vi "ScanDelay_FTIR_GetSpectrum_Aligning.vi"(0 "Cancel? External":refnum<vi>, 1 "% averaged (external)":refnum<vi>, 2 "Binned interferogram (external)":refnum<vi>, 3 "Python refnum in":refnum<k35>, 5 "Refresh alignment":bool=TRUE, 7 "Acquisition cycle (external)":refnum<vi>, 9 "Delay calibration\n          factor":dbl=2.403, 10 "Python error in":errorcluster, 11 "Subtract\ndelay (ps)":dbl, 12 "Acquisitions per interferogram":i32=20, 13 "Time per\nacquisition (s)":dbl=0.235, 14 "Sampling rate":dbl=250000.0, 15 "Extract envelope":bool=TRUE) -> (4 "Output spectrum":dbl[][](array[numeric]), 6 "Python error out":errorcluster)   [LabVIEW 2021]
uses:
  Control_GetSpectrum_Aligning.ctl
  <vilib>/DAQmx/read.llb/DAQmx Read (Analog 2D DBL NChan NSamp).vi
  <vilib>/DAQmx/miscellaneous.llb/DAQmx Fill In Error Info.vi
panel:
  out "DAQmx error":errorcluster={"status"=FALSE, "code"=200012, "source"="DAQmx Control Task.vi:3900001"}
  out "Time per\nloop (ms)":dbl=251.0
  in  "Save interferograms\n(interferograms.txt)":bool
  in  "Alignment order":i32=4
  out "Own python session":bool
  out "Refnum errors":errorcluster
  out "Spectrum (amplitude)":cluster{dbl[], dbl[]}[](graph)
  out "Spectrum (phase)":cluster{dbl[], dbl[]}(graph)
  out "Interferogram (aligned)":cluster{dbl, dbl}[](graph)
  out "% averaged":dbl=100.0
  out "Acquisition cycle":dbl[][](graph)
  in  "Halt acquisition":bool
  out "Python module path":path=path "C:/Users/mnopl/Desktop/Software/LabVIEW/ScanDelay/scandelay.py"
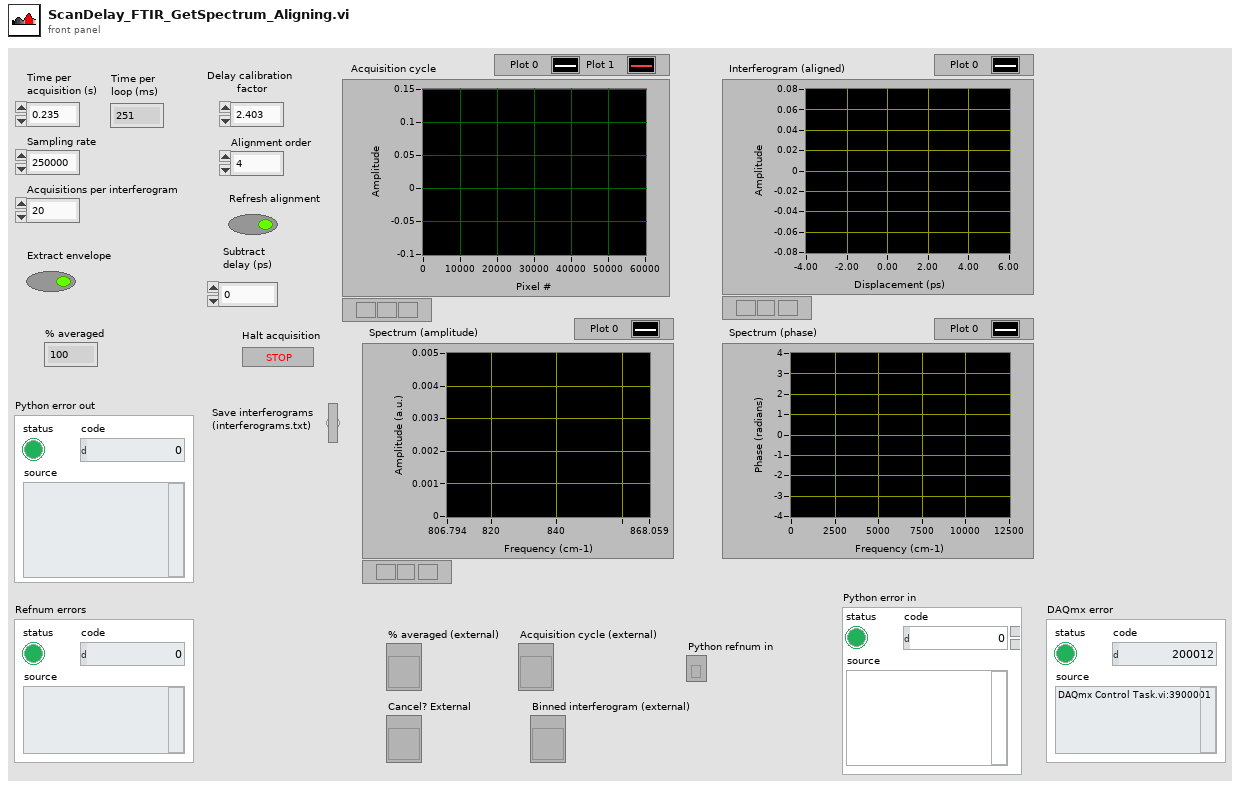
[diagram p1: front panel]
types:
  T1 = typedef "Control_GetSpectrum_Aligning.ctl" = enum16{"Acquire Interferograms", "Prepare DAQ task", "Align Interferograms", "Compute Spectrum", "Done"}
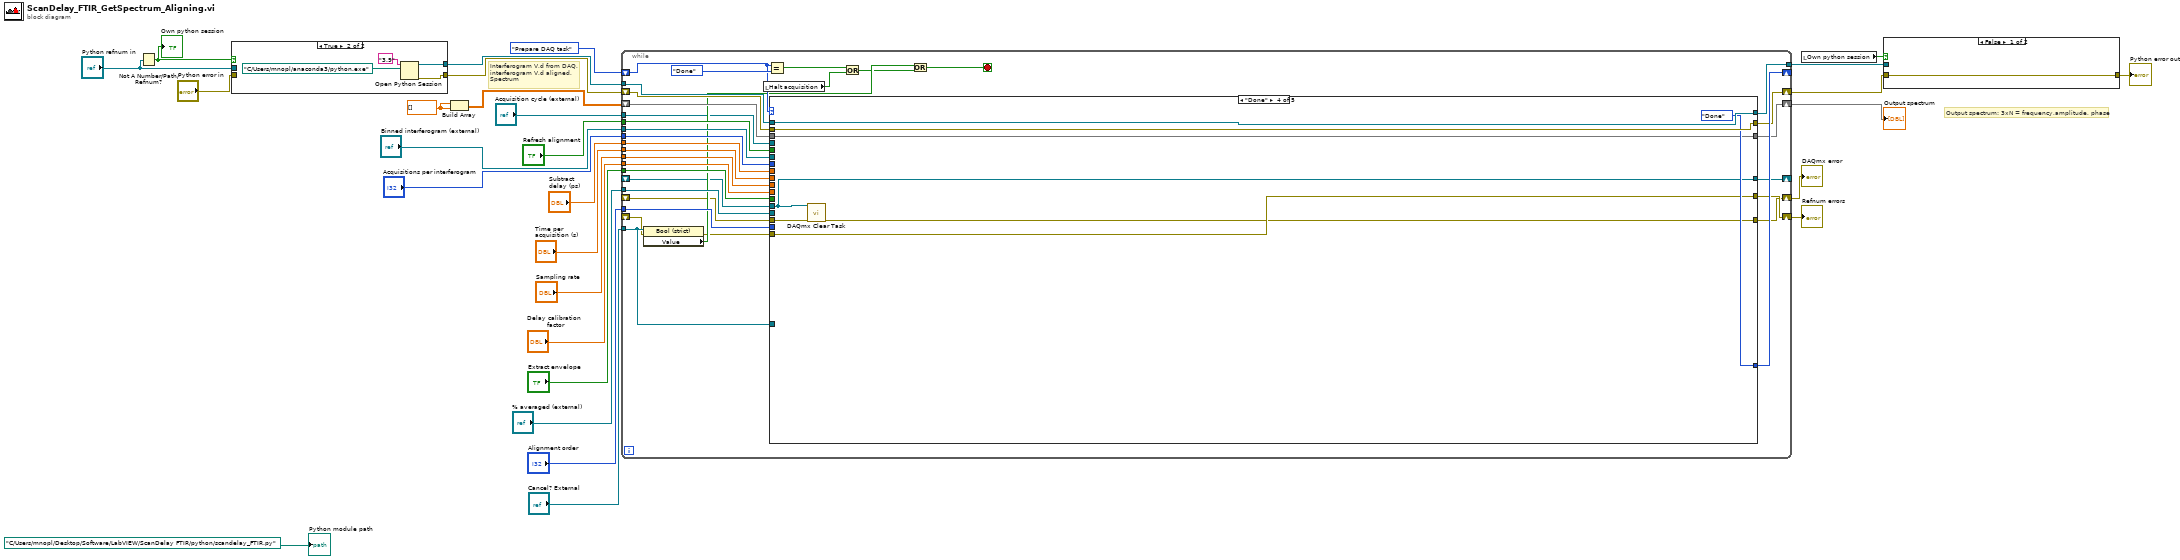
[diagram p0: block diagram]
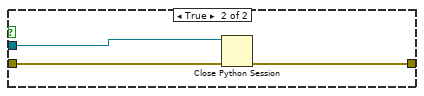
[diagram p2: hidden frame]
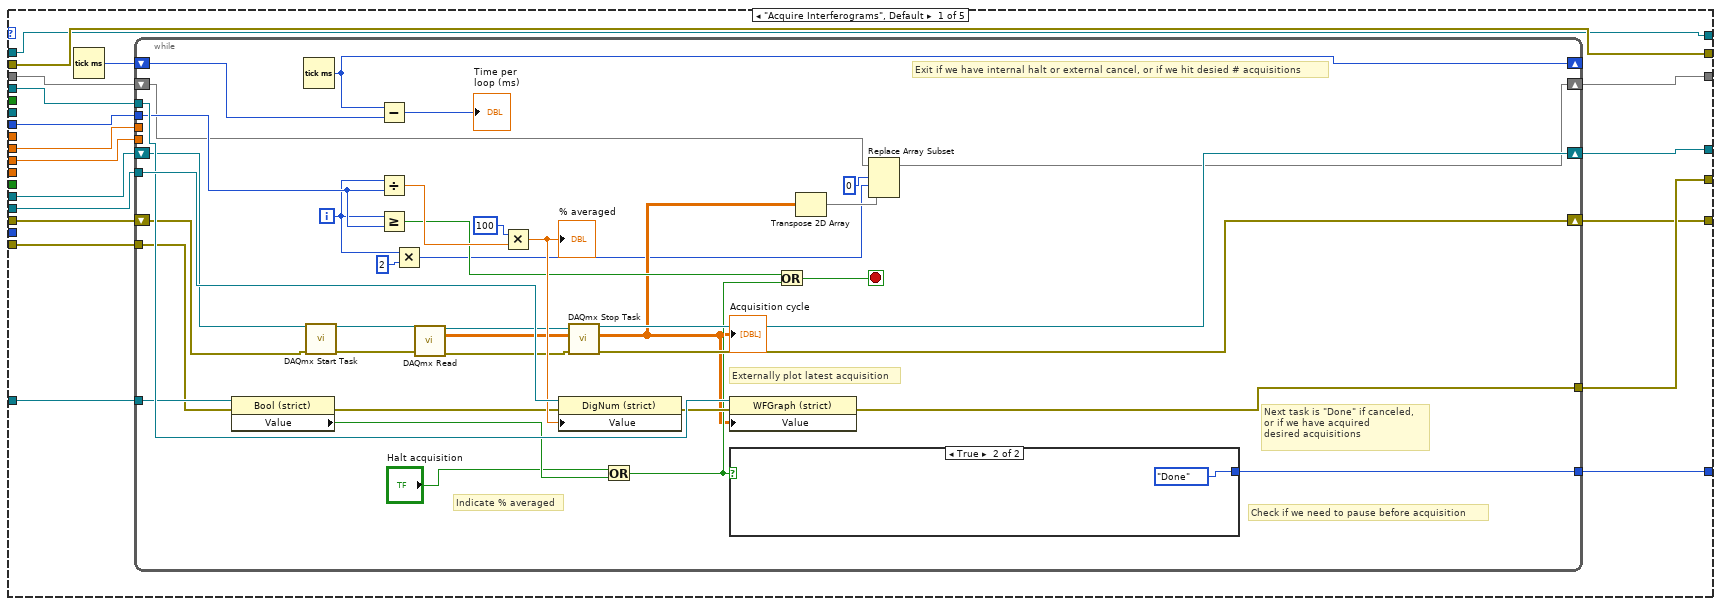
[diagram p4: hidden frame]
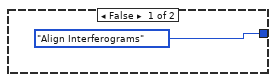
[diagram p5: hidden frame]
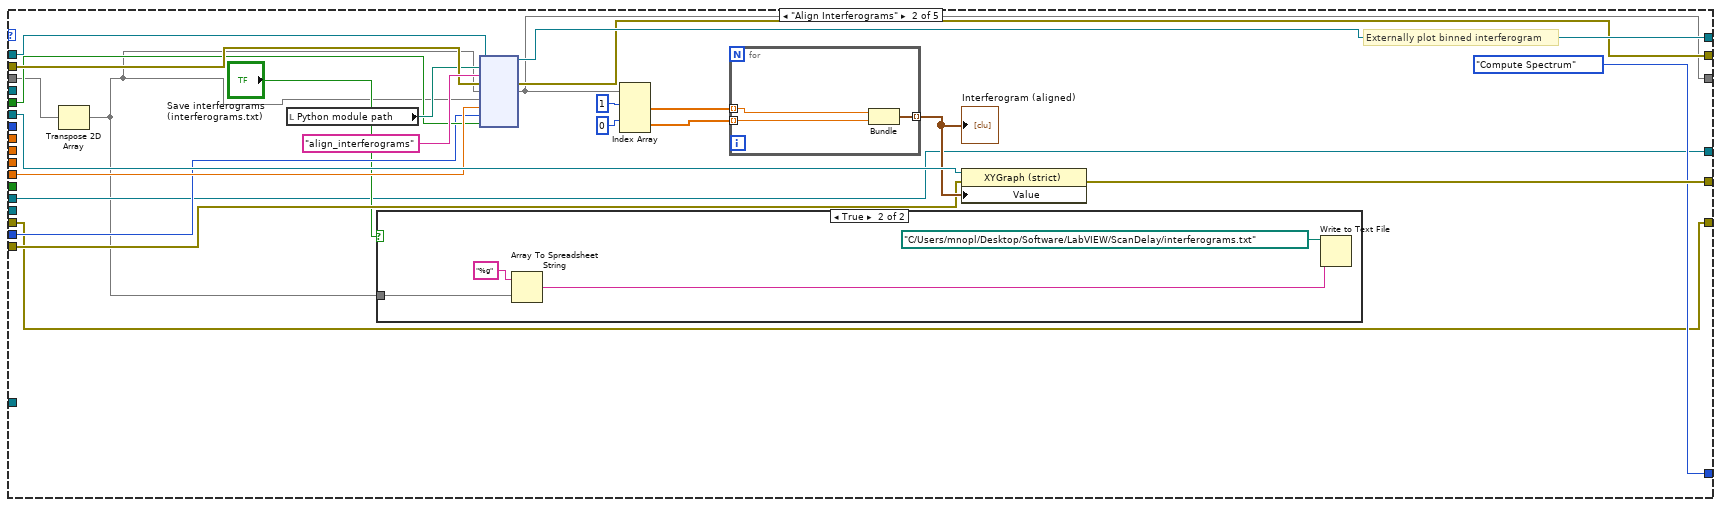
[diagram p6: hidden frame]
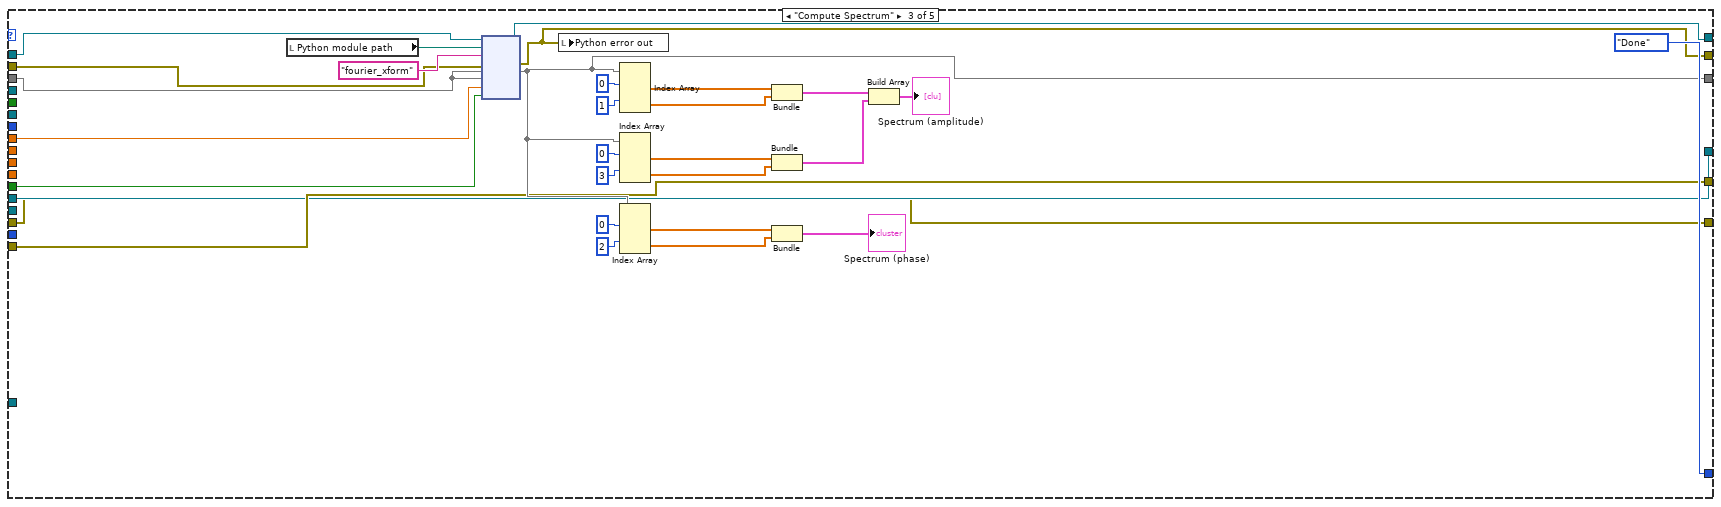
[diagram p8: hidden frame]
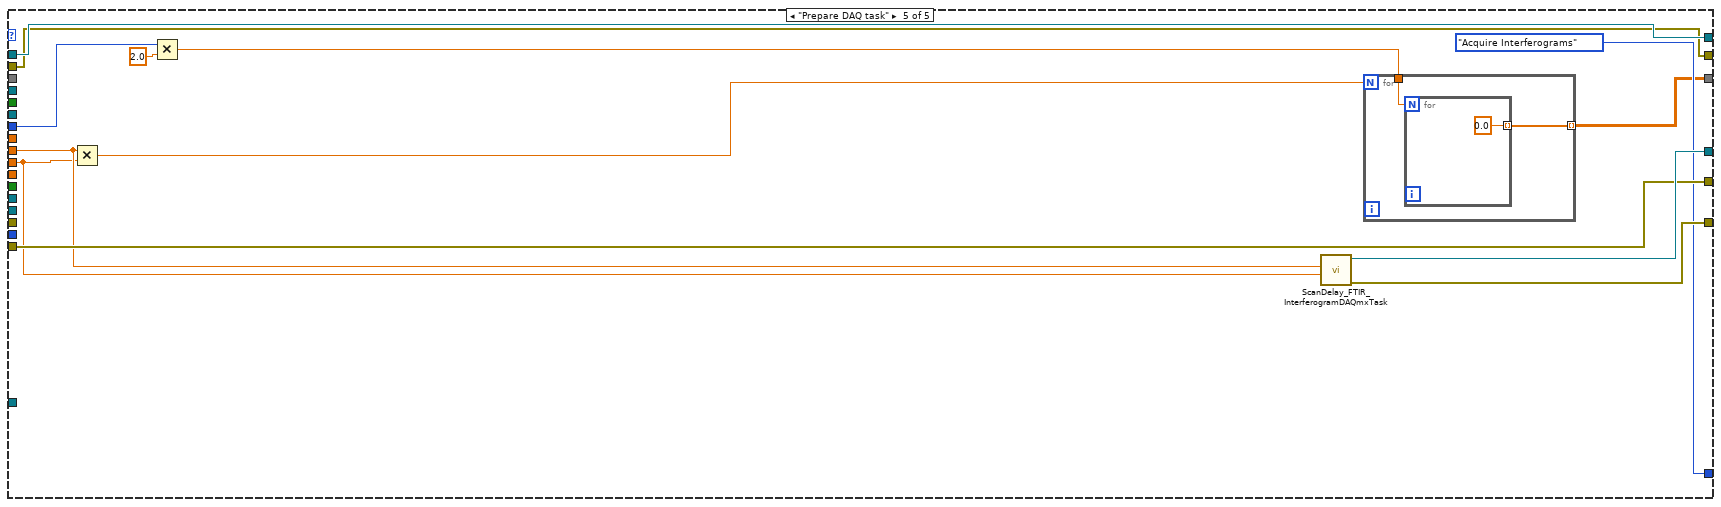
[diagram p9: hidden frame]
diagram:
  w17 = dbl[] []
  # "Output spectrum: 3xN = frequency,amplitude, phase"
  # "Interferogram V,d from DAQ,\ninterferogram V,d aligned,\nSpectrum"
  n1 = Not A Number/Path/Refnum?(number/path/refnum="Python refnum in") -> (NaN/Path/Refnum?=w7:bool)
  "Own python session" <- w7
  n2 = case shown="True" w7 {
    tunnel: [w30 w32] -> w11
    tunnel: [w29 w31] -> w10
    tunnel: "Python refnum in" -> [w30 _]
    tunnel: "Python error in" -> [w29 _]
    frame False {
    }
    frame True {
      n3 = Open Python Session(python version="3.9", python path=path "C:/Users/mnopl/anaconda3/python.exe") -> (session out=w32:refnum<k35>, error out=w31:errorcluster)  [unwired: 1 in]
    }
  }
  n4 = Build Array(w17, w17) -> (w4:dbl[][])
  n5 = while {
    shift-right: [w49] -> w16
    shift-left: w4 -> [w67]
    tunnel: w11 -> [w66]
    tunnel: "Acquisition cycle (external)" -> [w39]
    tunnel: "Sampling rate" -> [w64]
    tunnel: "Time per\nacquisition (s)" -> [w63]
    tunnel: "Delay calibration\n          factor" -> [w62]
    tunnel: "% averaged (external)" -> [w61]
    tunnel: "Cancel? External" -> [w42]
    tunnel: "Acquisitions per interferogram" -> [w60]
    shift-right: [w59] -> _
    shift-left: Control_GetSpectrum_Aligning."Prepare DAQ task" -> [w50]
    tunnel: "Subtract\ndelay (ps)" -> [w58]
    tunnel: [w55] -> w18
    shift-right: [w54] -> w15
    shift-left: w10 -> [w65]
    tunnel: "Extract envelope" -> [w53]
    shift-right: [w52] -> w13
    shift-left: _ -> [w40]
    tunnel: "Binned interferogram (external)" -> [w51]
    tunnel: "Refresh alignment" -> [w48]
    tunnel: "Alignment order" -> [w47]
    shift-right: [w37] -> w1
    shift-left: _ -> [w35]
    shift-right: [w38] -> _
    shift-left: _ -> [w36]
    stop <- w44 stop-if-true
    n6 = property on="Property Node" class="Bool (strict)"(reference=w42, error in=w40) -> (error out=w41:errorcluster, "Value"=w46:bool)  [unwired: 1 out]
    n7 = local read "Halt acquisition"() -> (w43:bool)
    n8 = Equal?(x=w50, y=Control_GetSpectrum_Aligning."Done") -> (x = y?=w56:bool)
    n9 = case shown="\"Done\"" w50 {
      tunnel: w67 -> [w68 w125 w183 w189 _]
      tunnel: w66 -> [w70 w146 w182 w191 w201]
      tunnel: w65 -> [w80 w145 w179 w192 w200]
      tunnel: w39 -> [w85 _ _ _ _]
      tunnel: w64 -> [w84 _ _ _ w195]
      tunnel: w63 -> [w83 _ _ _ w199]
      tunnel: w62 -> [_ w133 _ _ _]
      tunnel: w61 -> [w82 _ _ _ _]
      tunnel: w42 -> [w81 _ _ _ _]
      tunnel: w60 -> [w77 _ _ _ w196]
      tunnel: [w70 w144 w181 w191 w201] -> w55
      tunnel: [w75 Control_GetSpectrum_Aligning."Compute Spectrum" Control_GetSpectrum_Aligning."Done" Control_GetSpectrum_Aligning."Done" Control_GetSpectrum_Aligning."Acquire Interferograms"] -> w59
      tunnel: w58 -> [_ _ w178 _ _]
      tunnel: [w80 w140 w159 w192 w200] -> w54
      tunnel: w53 -> [_ _ w168 _ _]
      tunnel: [w79 w138 w157 w188 w203] -> w52
      tunnel: w51 -> [_ w139 _ _ _]
      tunnel: [w78 w132 w158 w189 w198] -> w49
      tunnel: w48 -> [_ w131 _ _ _]
      tunnel: w47 -> [_ w130 _ _ _]
      tunnel: w41 -> [w76 w129 w157 w188 w203]
      tunnel: [w72 w127 w156 w187 w205] -> w38
      tunnel: [w71 w126 w155 w185 w204] -> w37
      tunnel: w36 -> [w74 w127 w156 w187 _]
      tunnel: w35 -> [w73 w126 w155 w186 _]
      frame "Acquire Interferograms", Default {
        n10 = Tick Count (ms)() -> (millisecond timer value=w69:u32)
        n11 = while {
          tunnel: w85 -> [w117]
          tunnel: w84 -> [_]
          tunnel: w83 -> [_]
          tunnel: w82 -> [w119]
          tunnel: w81 -> [w114]
          tunnel: [w115] -> w79
          shift-right: [w99] -> w78
          shift-left: w68 -> [w98]
          tunnel: w77 -> [w108]
          tunnel: w76 -> [w113]
          tunnel: [w110] -> w75
          shift-right: [w105] -> w72
          shift-left: w74 -> [w88]
          shift-right: [w106] -> w71
          shift-left: w73 -> [w87]
          shift-right: [w104] -> _
          shift-left: w69 -> [w103]
          i -> [w101]
          stop <- w111 stop-if-true
          # "Next task is \"Done\" if canceled,\nor if we have acquired \ndesired acquisitions"
          # "Exit if we have internal halt or external cancel, or if we hit desied # acquisitions"
          # "Externally plot latest acquisition"
          # "Indicate % averaged"
          # "Check if we need to pause before acquisition"
          n12 = property on="Property Node" class="Bool (strict)"(reference=w114, error in=w113) -> (error out=w112:errorcluster, "Value"=w109:bool)  [unwired: 1 out]
          n13 = Tick Count (ms)() -> (millisecond timer value=w104:u32)
          n14 = call <vilib>:"DAQmx Start Task.vi"("task/channels in"=w88, "error in"=w87) -> ("task out"=w89:refnum<k21>, "error out"=w86:errorcluster)  [unwired: 12 in]
          n15 = Subtract(x=w104, y=w103) -> (x-y=→"Time per\nloop (ms)":u32)
          n16 = Divide(x=w101, y=w108) -> (x/y=w121:dbl)
          n17 = Greater Or Equal?(x=w101, y=w108) -> (x >= y?=w96:bool)
          n18 = Multiply(x=w101, y=2) -> (x*y=w92:i32)
          n19 = call-poly <vilib>:"DAQmx Read.vi"("task/channels in"=w89, "error in"=w86) -> ("task out"=w90:refnum<k21>, "data"=w94:dbl[][], "error out"=w107:errorcluster)  [unwired: 11 in]
          "Acquisition cycle" <- w94
          n20 = Multiply(x=100, y=w121) -> (x*y=w118:dbl)
          "% averaged" <- w118
          n21 = property on="Property Node" class="DigNum (strict)"(reference=w119, error in=w112, "Value"=w118) -> (error out=w116:errorcluster)  [unwired: 1 out]
          n22 = call <vilib>:"DAQmx Stop Task.vi"("task/channels in"=w90, "error in"=w107) -> ("task out"=w105:refnum<k21>, "error out"=w106:errorcluster)  [unwired: 12 in]
          n23 = Or(x="Halt acquisition", y=w109) -> (x .or. y?=w97:bool)
          n24 = property on="Property Node" class="WFGraph (strict)"(reference=w117, error in=w116, "Value"=w94) -> (error out=w115:errorcluster)  [unwired: 1 out]
          n25 = case shown="True" w97 {
            tunnel: [Control_GetSpectrum_Aligning."Align Interferograms" Control_GetSpectrum_Aligning."Done"] -> w110
            frame False {
            }
            frame True {
            }
          }
          n26 = Or(x=w96, y=w97) -> (x .or. y?=w111:bool)
          n27 = Transpose 2D Array(2D array=w94) -> (transposed array=w95:dbl[][])
          n28 = Replace Array Subset(array=w98, new element=w95, index (row)=0, index (col)=w92) -> (w99:dbl[][])
        }
      }
      frame "Align Interferograms" {
        # "Externally plot binned interferogram"
        n29 = Transpose 2D Array(2D array=w125) -> (transposed array=w124:dbl[][])
        n30 = local read "Python module path"() -> (w143:path)
        n31 = case shown="True" "Save interferograms\n(interferograms.txt)" {
          tunnel: w124 -> [_ w149]
          frame False {
          }
          frame True {
            n32 = Array To Spreadsheet String(array=w149, 3:"%g") -> (spreadsheet string=w151:string)  [unwired: 1 in]
            n33 = Write to Text File(file (use dialog)=path "C:/Users/mnopl/Desktop/Software/LabVIEW/ScanDelay/interferograms.txt", text=w151) -> ()  [unwired: 2 in, 3 out]
          }
        }
        n34 = node(w146, w143, "align_interferograms", w145, w124, w124, w133, w130, w131) -> (w144:refnum<k35>, w140:errorcluster, w132:dbl[][])  [unwired: 4 in, 2 out]
        n35 = Index Array(array=w132, index (row) #1=1, index (row) #2=0) -> (element #1=w136:dbl[], element #2=w137:dbl[])  [unwired: 2 in]
        n36 = for {
          tunnel: w137 -> [w153] mode=indexing
          tunnel: w136 -> [w154] mode=indexing
          tunnel: [w152] -> w135 mode=indexing
          n37 = Bundle(w154, w153) -> (w152:cluster{dbl, dbl})  [unwired: 1 in]
        }
        "Interferogram (aligned)" <- w135
        n38 = property on="Property Node" class="XYGraph (strict)"(reference=w139, error in=w129, "Value"=w135) -> (error out=w138:errorcluster)  [unwired: 1 out]
      }
      frame "Compute Spectrum" {
        n39 = local read "Python module path"() -> (w180:path)
        n40 = node(w182, w180, "fourier_xform", w179, w183, w183, w178, w168) -> (w181:refnum<k35>, w159:errorcluster, w158:dbl[][])  [unwired: 3 in, 2 out]
        n41 = local write "Python error out"(w159) -> ()
        n42 = Index Array(array=w158, index (row) #1=0, index (row) #2=1) -> (element #1=w174:dbl[], element #2=w173:dbl[])  [unwired: 2 in]
        n43 = Index Array(array=w158, index (row) #1=0, index (row) #2=3) -> (element #1=w169:dbl[], element #2=w170:dbl[])  [unwired: 2 in]
        n44 = Index Array(array=w158, index (row) #1=0, index (row) #2=2) -> (element #1=w164:dbl[], element #2=w165:dbl[])  [unwired: 2 in]
        n45 = Bundle(w174, w173) -> (w162:cluster{dbl[], dbl[]})  [unwired: 1 in]
        n46 = Bundle(w169, w170) -> (w161:cluster{dbl[], dbl[]})  [unwired: 1 in]
        n47 = Bundle(w164, w165) -> (→"Spectrum (phase)":cluster{dbl[], dbl[]})  [unwired: 1 in]
        n48 = Build Array(w162, w161) -> (→"Spectrum (amplitude)":cluster{dbl[], dbl[]}[])
      }
      frame "Done" {
        n49 = call <vilib>:"DAQmx Clear Task.vi"("task in"=w187, "error in"=w186) -> ("error out"=w185:errorcluster)  [unwired: 13 in]
      }
      frame "Prepare DAQ task" {
        n50 = Multiply(x=w199, y=w195) -> (x*y=w194:dbl)
        n51 = Multiply(x=w196, y=2.0) -> (x*y=w193:dbl)
        n52 = call "ScanDelay_FTIR_InterferogramDAQmxTask.vi"("Sampling rate"=w195, "Time per acquisiton (s)"=w199) -> ("error out"=w204:errorcluster, "Refnum out"=w205:refnum<k21>)  [unwired: 8 in]
        n53 = for {
          N: w194 -> [_]
          tunnel: [w207] -> w198 mode=indexing
          tunnel: w193 -> [w206]
          n54 = for {
            N: w206 -> [_]
            tunnel: [0.0] -> w207 mode=indexing
          }
        }
      }
    }
    n55 = Or(x=w56, y=w43) -> (x .or. y?=w45:bool)
    n56 = Or(x=w46, y=w45) -> (x .or. y?=w44:bool)
  }
  "Output spectrum" <- w16
  "Refnum errors" <- w13
  "DAQmx error" <- w1
  n57 = local read "Own python session"() -> (w6:bool)
  n58 = case shown="False" w6 {
    tunnel: [w209 w212] -> w19
    tunnel: w18 -> [_ w211]
    tunnel: w15 -> [w209 w210]
    frame False {
    }
    frame True {
      n59 = Close Python Session(session in=w211, error in=w210) -> (11:w212:errorcluster)
    }
  }
  "Python error out" <- w19
  "Python module path" <- path "C:/Users/mnopl/Desktop/Software/LabVIEW/ScanDelay FTIR/python/scandelay_FTIR.py"
